vi "reconnect.vi"(8 "error in (no error)":errorcluster, 11 "MonoClientCommunicator in":refnum<class "MonoClientCommunicator.lvclass">) -> (0 "error out":errorcluster, 3 "MonoClientCommunicator out":refnum<class "MonoClientCommunicator.lvclass">)   [LabVIEW 2016, in "MonoClientCommunicator.lvclass"]
uses:
  MonoClientCommunicator.lvclass
  MonoClientCommunicator.lvclass/MonoClientCommunicator.ctl
  ts_labview_tcp/TCPClient/TCPClient.lvclass
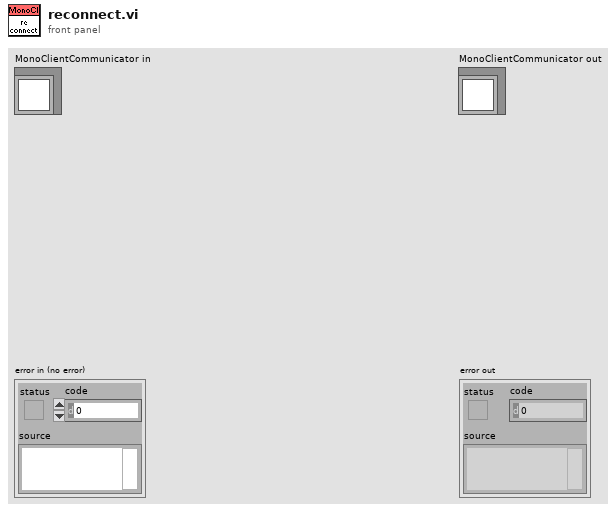
[diagram p1: front panel]
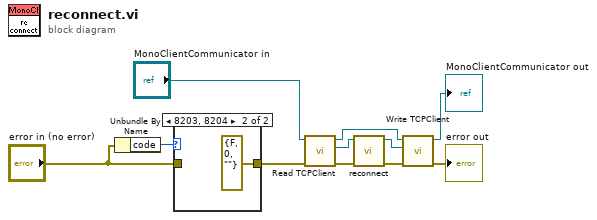
[diagram p0: block diagram]
diagram:
  n1 = Unbundle By Name("error in (no error)") -> ("code"=w3:i32)
  n2 = case shown="8203, 8204" w3 {
    tunnel: [w12 errorcluster {"status"=FALSE, "code"=0, "source"=""} ("error in (no error)")] -> w2
    tunnel: "error in (no error)" -> [w12 _]
    frame 0, Default {
    }
    frame 8203, 8204 {
    }
  }
  n3 = call "Read TCPClient.vi"("error in (no error)"=w2, "MonoClient in"="MonoClientCommunicator in") -> ("error out"=w4:errorcluster, "TCPClient.lvclass"=w7:refnum<class "TCPClient.lvclass">, "MonoClient out"=w11:refnum<class "MonoClientCommunicator.lvclass">)  [unwired: 7 in]
  n4 = call-dynamic "reconnect.vi"("error in (no error)"=w4, "TCPCommunicator in"=w7) -> ("error out"=w5:errorcluster, "TCPCommunicator out"=w6:refnum<class "TCPClient.lvclass">)  [unwired: 8 in]
  n5 = call "Write TCPClient.vi"("error in (no error)"=w5, "TCPClient.lvclass"=w6, "MonoClient in"=w11) -> ("error out"=→"error out":errorcluster, "MonoClient out"=→"MonoClientCommunicator out":refnum<class "MonoClientCommunicator.lvclass">)  [unwired: 7 in]
